vi "Cryo-Con check complete.vi"(8 "Error In":errorcluster, 11 "VISA resource name":refnum<visa-resource-name>) -> (0 "Error Out":errorcluster, 3 "VISA resource name out":refnum<visa-resource-name>)   [LabVIEW 2015]
uses:
  GPIB/VISA  Send Receive.vi
panel:
  out "Array":string[](array[string])
  out "data string out":string
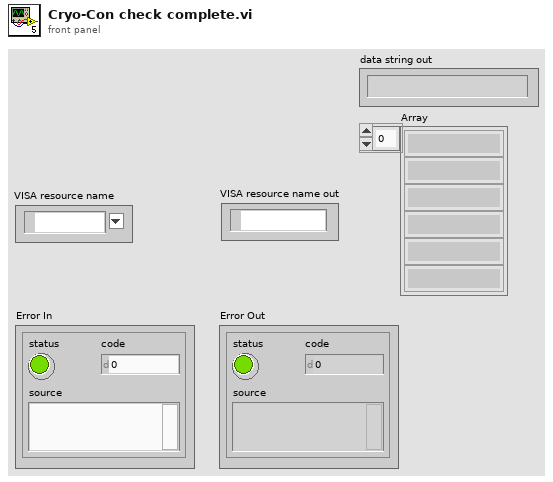
[diagram p1: front panel]
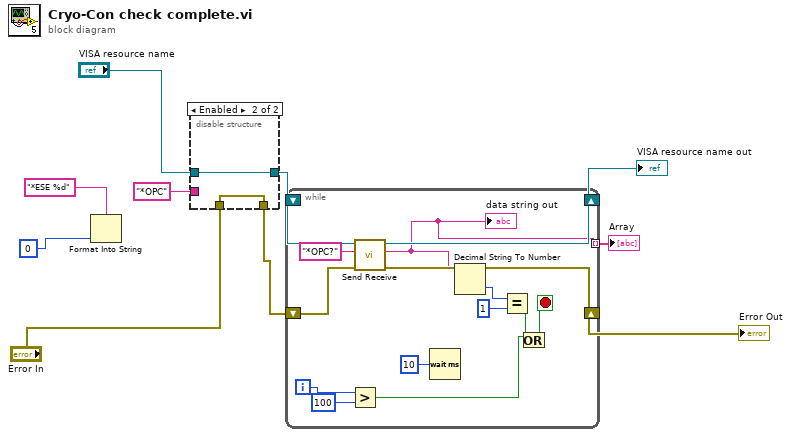
[diagram p0: block diagram]
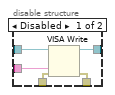
[diagram p2: hidden frame]
diagram:
  n1 = Format Into String(format string="*ESE %d", 0) -> ()  [unwired: 2 in, 2 out]
  n2 = disable-structure shown="Enabled" {
    disable-tunnel: "VISA resource name" -> [w15 w16]
    disable-tunnel: [w14 w16] -> w7
    disable-tunnel: "Error In" -> [w13 w17]
    disable-tunnel: [w12 w17] -> w5
    disable-tunnel: "*OPC" ("write buffer") -> [w11 _]
    frame Disabled {
      n3 = VISA Write(VISA resource name=w15, write buffer=w11, error in (no error)=w13) -> (VISA resource name out=w14:refnum<visa-resource-name>, error out=w12:errorcluster)  [unwired: 1 out]
    }
    frame Enabled {
    }
  }
  n4 = while {
    shift-right: [w31] -> w9
    shift-left: w7 -> [w28]
    shift-right: [w30] -> w8
    shift-left: w5 -> [w27]
    tunnel: [w18] -> w1 mode=indexing
    i -> [w22]
    stop <- w20 stop-if-true
    n5 = Greater?(x=w22, y=100) -> (0:w19:bool)
    n6 = call-poly "Send Receive.vi"("error in (no error)"=w27, "data string in"="*OPC?", "VISA Resource Name"=w28) -> ("error out"=w30:errorcluster, "data string out"=w18:string, "VISA Resource Name Out"=w31:refnum<visa-resource-name>)  [unwired: 6 in]
    "data string out" <- w18
    n7 = Wait (ms)(milliseconds to wait=u32 10) -> ()  [unwired: 1 out]
    n8 = Decimal String To Number(string=w18) -> (number=w26:i32)  [unwired: 2 in, 1 out]
    n9 = Equal?(x=w26, y=1) -> (x = y?=w24:bool)
    n10 = Or(x=w19, y=w24) -> (x .or. y?=w20:bool)
  }
  "Error Out" <- w8
  "VISA resource name out" <- w9
  "Array" <- w1
